vi "Resources.vi"() -> (3 "Resources":refnum<class "VisaResource.lvclass">[](array[class]))   [LabVIEW 2020, in "RP2040.lvlib" / "RP2040Target.lvclass"]
uses:
  RP2040Target.lvclass
  VisaResource/VisaResource.lvclass
  <vilib>/Instr/_visa.llb/VISA Find Search Mode.ctl
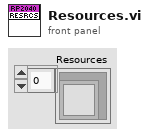
[diagram p1: front panel]
types:
  T1 = typedef "VISA Find Search Mode.ctl" = u32
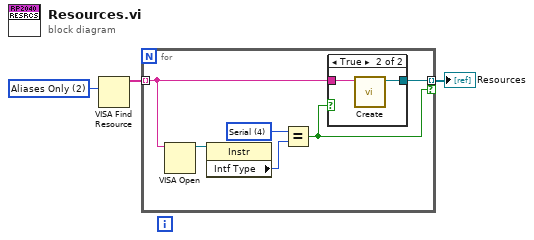
[diagram p0: block diagram]
diagram:
  w3 = T1 2 items=["Canonical Names Only"=0, "Aliases Only"=2, "Include Matching Aliases"=3, "Include All Aliases"=4] ("Search Mode")
  n1 = VISA Find Resource(10:w3) -> (3:w2:string[])  [unwired: 2 in, 2 out]
  n2 = for {
    tunnel: w2 -> [w8] mode=indexing
    tunnel: [w9] -> w1 mode=indexing if=w4
    w6 = u16 4 items=["GPIB"=1, "VXI"=2, "GPIB-VXI"=3, "Serial"=4, "PXI"=5, "TCPIP"=6, "USB"=7, "FireWire"=9] ("Interface Information:Interface Type")
    n3 = VISA Open(VISA resource name=w8) -> (VISA resource name=w7:refnum<visa-resource-name>)  [unwired: 4 in, 1 out]
    n4 = property class="Instr"(reference=w7) -> ("Intf Type"=w5:u16)  [unwired: 1 in, 2 out]
    n5 = Equal?(x=w6, y=w5) -> (x = y?=w4:bool)
    n6 = case shown="True" w4 {
      tunnel: [_ w11] -> w9
      tunnel: w8 -> [_ w10]
      frame False {
      }
      frame True {
        n7 = call "Create.vi"("Port"=w10) -> ("VisaResource out"=w11:refnum<class "VisaResource.lvclass">)  [unwired: 9 in, 1 out]
      }
    }
  }
  "Resources" <- w1
